vi "FTW-TestExecutive-Core_StepTypes_Definitions.vi"(0 "FTW-TestExecutive-Core In":refnum<class "FTW-TestExecutive-Core.lvclass">, 11 "error in":errorcluster) -> (4 "FTW-TestExecutive-Core Out":refnum<class "FTW-TestExecutive-Core.lvclass">, 8 "Step Types":cluster{"Name":string, "Base Config":string}[](array[cluster]), 15 "error out":errorcluster)   [LabVIEW 2015, in "FTW-TestExecutive-Core.lvclass"]
uses:
  FTW-TestExecutive-Core.lvclass
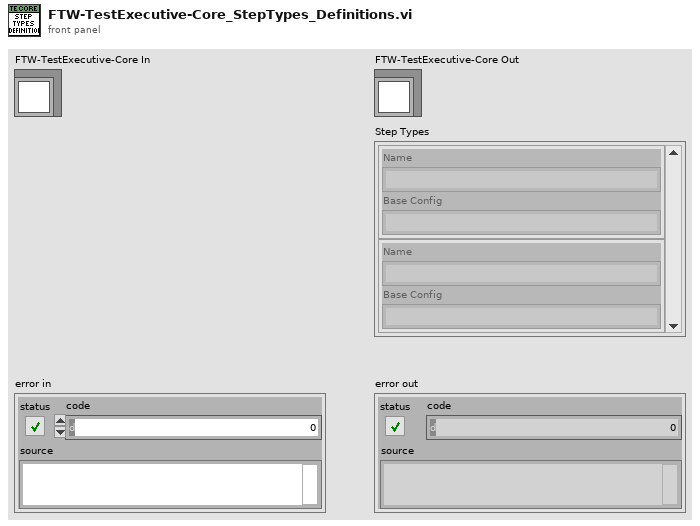
[diagram p1: front panel]
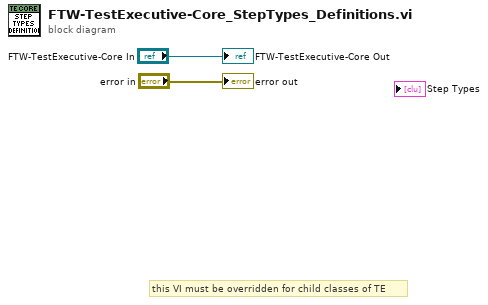
[diagram p0: block diagram]
diagram:
  # "this VI must be overridden for child classes of TE"
  "FTW-TestExecutive-Core Out" <- "FTW-TestExecutive-Core In"
  "error out" <- "error in"
